vi "NanoGauge.vi"() -> ()   [LabVIEW 2012]
uses:
  Madlib.dll
panel:
  in  "Results File":path
  out "Milliseconds":i32
  in  "Time Spacing (ms)":i32
  in  "Averages":u16=1 min=1 step=1
  out "Encoder Position (um)":dbl(graph)
  in  "?":bool
  in  "?":bool
  out "Position um":dbl min=0.0 max=100.0 step=0.001 format="%.4f"
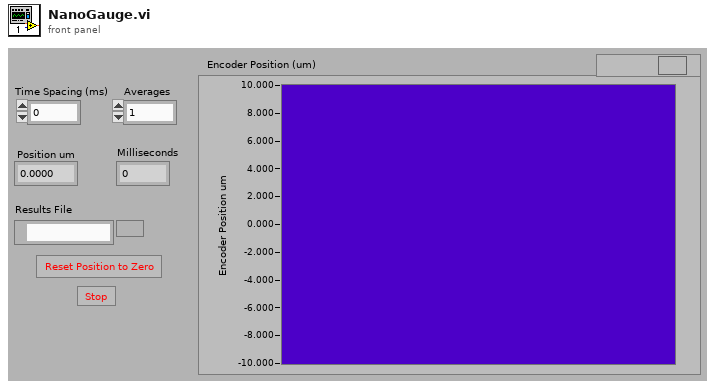
[diagram p1: front panel]
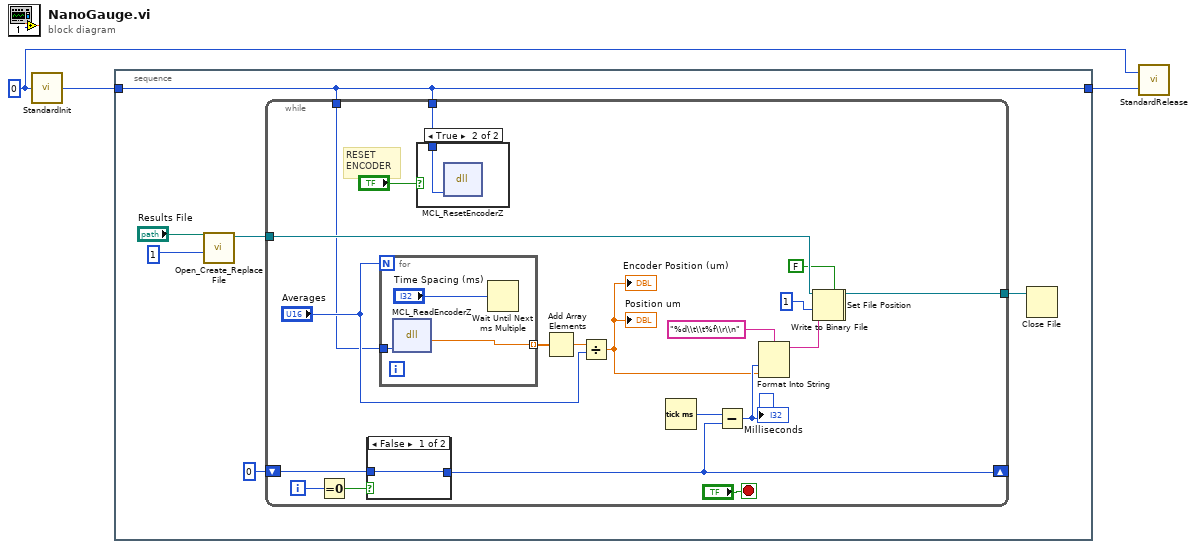
[diagram p0: block diagram]
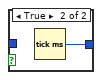
[diagram p2: hidden frame]
diagram:
  w2 = 0
  n1 = call "StandardInit.vi"("Incoming Handle"=w2) -> ("Outgoing Handle"=w3:i32)
  n2 = stacked-sequence {
    tunnel: w3 -> [w4]
    tunnel: [w4] -> w1
    frame #0 {
      n3 = call <vilib>:"Open_Create_Replace File.vi"("function (open:0)"=1, "file path"="Results File") -> ("refnum"=w6:refnum<file>)  [unwired: 6 in, 3 out]
      n4 = while {
        shift-right: [w22] -> _
        shift-left: 0 -> [w24]
        tunnel: w6 -> [w20]
        tunnel: [w19] -> w5
        tunnel: w4 -> [w14]
        tunnel: w4 -> [w13]
        i -> [w26]
        stop <- "?" stop-if-true
        # "RESET\nENCODER"
        n5 = Equal To 0?(x=w26) -> (x = 0?=w25:bool)
        n6 = case shown="False" w25 {
          tunnel: [w32 w33] -> w22
          tunnel: w24 -> [w32 _]
          frame False {
          }
          frame True {
            n7 = Tick Count (ms)() -> (millisecond timer value=w33:u32)
          }
        }
        n8 = for {
          N: "Averages" -> [_]
          tunnel: [w34] -> w29 mode=indexing
          tunnel: w13 -> [w35]
          n9 = dll-call lib="C:/Users/Labview/Desktop/SRR/Madlib_x64/Labview Examples/MADLib.dll" fn="MCL_ReadEncoderZ"("handle"=w35) -> (w34:dbl)  [unwired: 4 in, 2 out]
          n10 = Wait Until Next ms Multiple(millisecond multiple="Time Spacing (ms)") -> ()  [unwired: 1 out]
        }
        n11 = case shown="True" "?" {
          tunnel: w14 -> [_ w37]
          frame False {
          }
          frame True {
            n12 = dll-call lib="C:/Users/Labview/Desktop/SRR/Madlib_x64/Labview Examples/MADLib.dll" fn="MCL_ResetEncoderZ"("handle"=w37) -> ()  [unwired: 5 in, 2 out]
          }
        }
        n13 = Add Array Elements(numeric array=w29) -> (sum=w28:dbl)
        n14 = Divide(x=w28, y="Averages") -> (x/y=w17:dbl)
        "Encoder Position (um)" <- w17
        "Position um" <- w17
        n15 = Tick Count (ms)() -> (millisecond timer value=w23:u32)
        n16 = Subtract(x=w23, y=w22) -> (x-y=w18:u32)
        "Milliseconds" <- w18
        n17 = Format Into String(format string="%d\\t\\t%f\\r\\n", w18, w17) -> (resulting string=w15:string)  [unwired: 2 in, 1 out]
        n18 = Set File Position(refnum=w20, from (0:start)=1) -> (refnum out=w12:refnum<file>, error out=w11:errorcluster)  [unwired: 2 in]
        n19 = Write to Binary File(file (use dialog)=w12, data=w15, error in=w11, 5:FALSE ("prepend array or string size? (T)")) -> (refnum out=w19:refnum<file>)  [unwired: 2 in, 2 out]
      }
      n20 = Close File(refnum=w5) -> ()  [unwired: 1 in, 2 out]
    }
  }
  n21 = call "StandardRelease.vi"("Outgoing Handle"=w1, "Incoming Handle"=w2) -> ()  [unwired: 1 in]
